vi "setHeatSpotLocations(SubVI).vi"(4 "YValue":dbl, 6 "XValue":dbl, 7 "Index":dbl, 8 "Set active":bool) -> ()   [LabVIEW 2020]
uses:
  <vilib>/httpClient/POSTBuffer.vi
  <vilib>/httpClient/LabVIEWHTTPClient.lvlib
panel:
  out "body 3":string
  out "body 2":string
  out "body":string
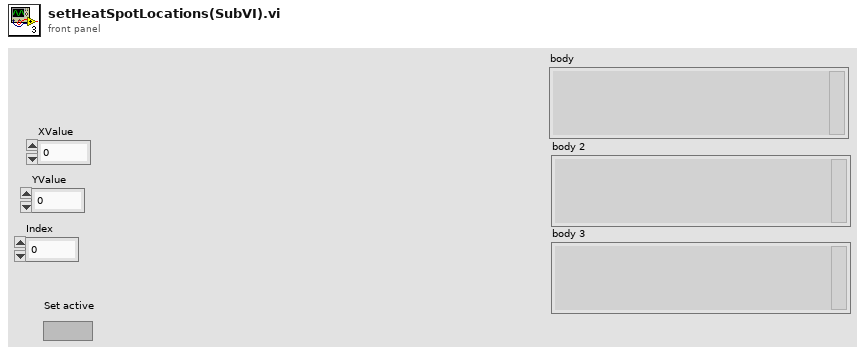
[diagram p1: front panel]
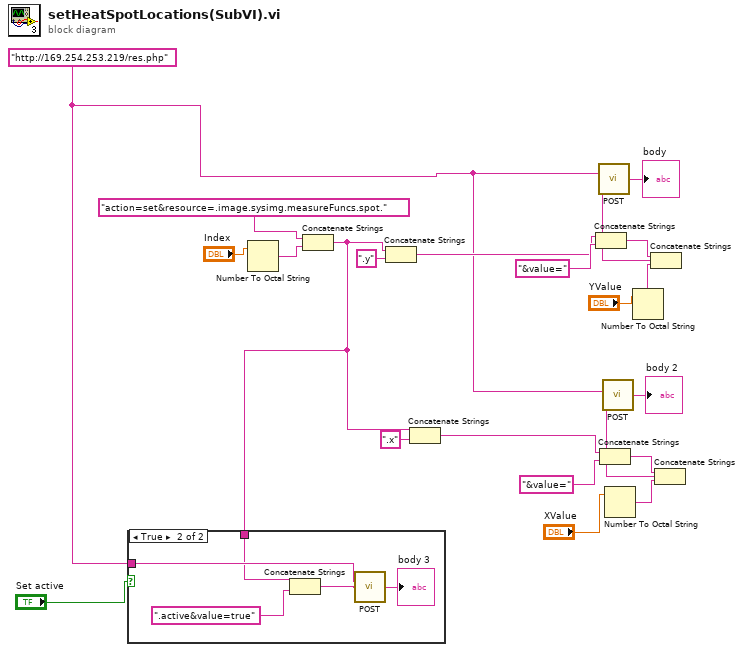
[diagram p0: block diagram]
diagram:
  w5 = "http://169.254.253.219/res.php" ("url")
  n1 = Number To Octal String(2:"Index") -> (0:w16:string)  [unwired: 1 in]
  n2 = Concatenate Strings("action=set&resource=.image.sysimg.measureFuncs.spot." ("buffer"), w16) -> (w4:string)
  n3 = case shown="True" "Set active" {
    tunnel: w5 -> [_ w27]
    tunnel: w4 -> [_ w26]
    frame False {
    }
    frame True {
      n4 = Concatenate Strings(w26, ".active&value=true" ("buffer")) -> (w24:string)
      n5 = call-poly <vilib>:"POST.vi"("url"=w27, "buffer"=w24) -> ("body"=→"body 3":string)  [unwired: 10 in, 3 out]
    }
  }
  n6 = Concatenate Strings(w4, ".y" ("string")) -> (w13:string)
  n7 = Concatenate Strings(w4, ".x" ("string")) -> (w12:string)
  n8 = Concatenate Strings(w13, "&value=" ("buffer")) -> (w21:string)
  n9 = Concatenate Strings(w12, "&value=" ("buffer")) -> (w8:string)
  n10 = Number To Octal String(2:"XValue") -> (0:w9:string)  [unwired: 1 in]
  n11 = Number To Octal String(2:"YValue") -> (0:w19:string)  [unwired: 1 in]
  n12 = Concatenate Strings(w21, w19) -> (w18:string)
  n13 = call-poly <vilib>:"POST.vi"("url"=w5, "buffer"=w18) -> ("body"=→"body":string)  [unwired: 10 in, 3 out]
  n14 = Concatenate Strings(w8, w9) -> (w10:string)
  n15 = call-poly <vilib>:"POST.vi"("url"=w5, "buffer"=w10) -> ("body"=→"body 2":string)  [unwired: 10 in, 3 out]
